vi "format_fridge_valve_data.vi"(9 "value_adc":dbl, 10 "value_motor":dbl, 11 "time":timestamp) -> (3 "waveform_array":waveform(dbl)[](array[waveform]))   [LabVIEW 2019]
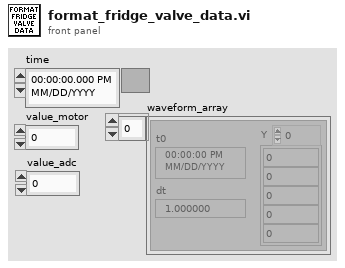
[diagram p1: front panel]
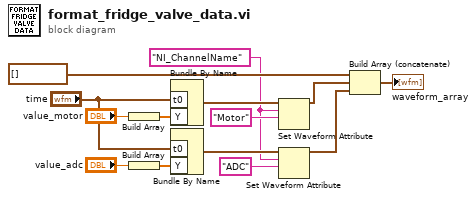
[diagram p0: block diagram]
diagram:
  w4 = "NI_ChannelName" ("name")
  n1 = Build Array("value_motor") -> (w13:dbl[])
  n2 = Build Array("value_adc") -> (w8:dbl[])
  n3 = Bundle By Name("t0"="time", "Y"=w13) -> (w11:waveform(dbl))  [unwired: 1 in]
  n4 = Bundle By Name("t0"="time", "Y"=w8) -> (w7:waveform(dbl))  [unwired: 1 in]
  n5 = Set Waveform Attribute(5:"Motor", 6:w4, 7:w11) -> (3:w12:waveform(dbl))  [unwired: 1 in, 2 out]
  n6 = Set Waveform Attribute(5:"ADC", 6:w4, 7:w7) -> (3:w2:waveform(dbl))  [unwired: 1 in, 2 out]
  n7 = Build Array (concatenate)(waveform(dbl)[] [], w12, w2) -> (→"waveform_array":waveform(dbl)[])
